vi "Set View Size.vi"(8 "error in (no error)":errorcluster, 10 "TabDimension":T1={"Width"=96, "Height"=200}, 11 "TabControlRef in":refnum<vi>) -> (0 "error out":errorcluster, 3 "TabControlRef out":refnum<vi>)   [LabVIEW 2020, in "MDI ViewManager.lvlib"]
uses:
  MDI ViewManager.lvlib
  <vilib>/Utility/miscctls.llb/LVBoundsTypeDef.ctl
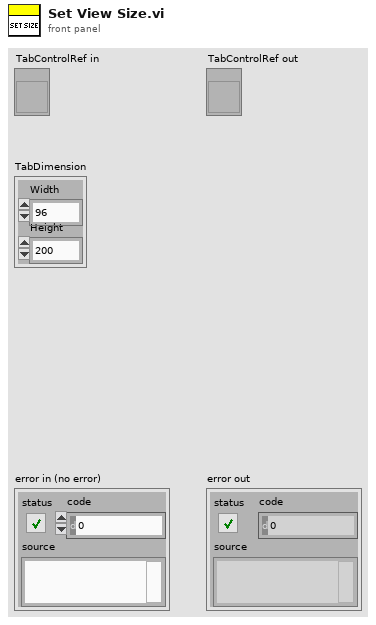
[diagram p1: front panel]
types:
  T1 = typedef "LVBoundsTypeDef.ctl" = cluster{"Width":u32, "Height":u32}
  T2 = typedef "LVPositionTypeDef.ctl" = cluster{"Left":i32, "Top":i32}
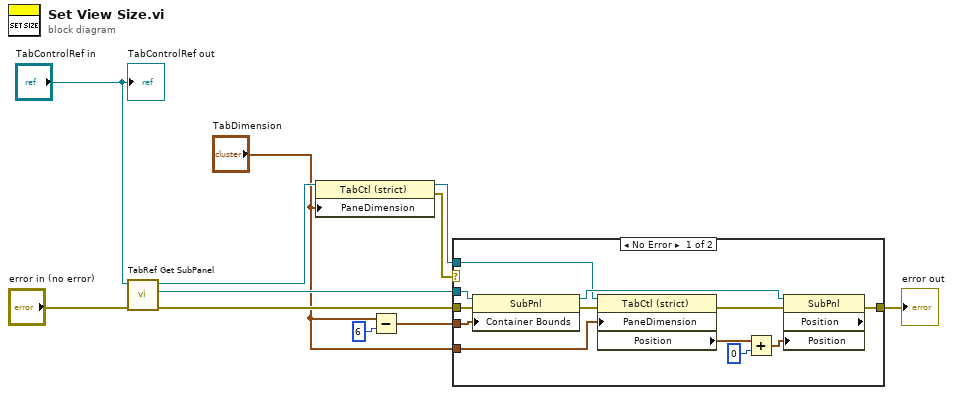
[diagram p0: block diagram]
diagram:
  n1 = call "TabRef Get SubPanel.vi"("error in (no error)"="error in (no error)", "TabControl in"="TabControlRef in") -> ("error out"=w10:errorcluster, "Sub Panel"=w11:refnum<vi>, "TabControl out"=w7:refnum<vi>)  [unwired: 7 in]
  n2 = property class="TabCtl (strict)"(reference=w7, "PaneDimension"="TabDimension") -> (reference out=w3:refnum<vi>, error out=w6:errorcluster)  [unwired: 1 in]
  n3 = Subtract(x="TabDimension", y=6) -> (x-y=w8:T1)
  n4 = case shown="No Error" w6 {
    selector: w6 -> [_ w24]
    tunnel: w11 -> [w23 _]
    tunnel: w10 -> [w21 _]
    tunnel: w8 -> [w16 _]
    tunnel: w3 -> [w15 _]
    tunnel: "TabDimension" -> [w14 _]
    tunnel: [w13 w24] -> w5
    frame No Error {
      n5 = property class="SubPnl"(reference=w23, error in=w21, "Container Bounds"=w16) -> (reference out=w20:refnum<vi>, error out=w22:errorcluster)
      n6 = property class="TabCtl (strict)"(reference=w15, error in=w22, "PaneDimension"=w14) -> (error out=w19:errorcluster, "Position"=w18:T2)  [unwired: 1 out]
      n7 = Add(x=w18, y=0) -> (x+y=w17:T2)
      n8 = property class="SubPnl" props=["Position", "Position"](reference=w20, error in=w19, "Position"=w17) -> (error out=w13:errorcluster)  [unwired: 2 out]
    }
    frame Error {
    }
  }
  "error out" <- w5
  "TabControlRef out" <- "TabControlRef in"
